vi "PWM_Default_Values.vi"() -> (3 "PWM_default":cluster{"High (uSec)":u32, "Period (uSec)":u32})   [LabVIEW 2009, in "PWM.lvlib"]
uses:
  PWM.lvlib
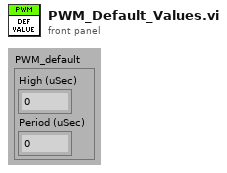
[diagram p1: front panel]
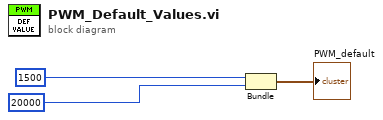
[diagram p0: block diagram]
diagram:
  n1 = Bundle("High (uSec)"=u32 1500, "Period (uSec)"=u32 20000) -> (→"PWM_default":cluster{"High (uSec)":u32, "Period (uSec)":u32})  [unwired: 1 in]
